vi "variable_stop_globale.vi"() -> ()   [LabVIEW 2017]
panel:
  out "stop":bool
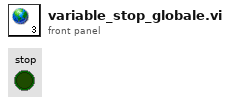
[diagram p1: front panel]
diagram:
